vi "picoquant_enqueue_loop_queue.vi"(8 "error in (no error)":errorcluster, 10 "element":T1, 11 "picoquant_generic in":refnum<class "picoquant_generic.lvclass">) -> (0 "error out":errorcluster, 3 "picoquant_generic out":refnum<class "picoquant_generic.lvclass">)   [LabVIEW 2015, in "picoquant_generic.lvclass"]
uses:
  picoquant_generic.lvclass
  loop_notifier_tdef.ctl
  picoquant_generic.lvclass/picoquant_generic.ctl
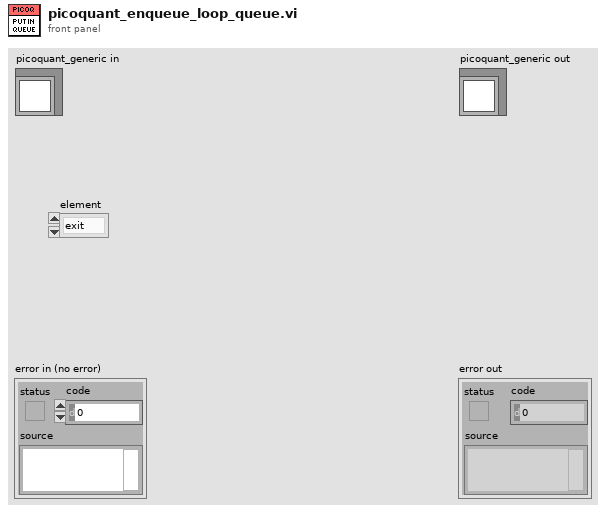
[diagram p1: front panel]
types:
  T1 = typedef "loop_notifier_tdef.ctl" = enum16{"exit"}
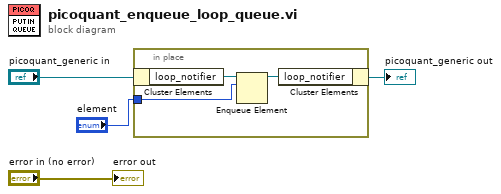
[diagram p0: block diagram]
diagram:
  n1 = in-place {
    in-place-border: "element" -> [w5]
    n2 = in-place-cluster #1("picoquant_generic in") -> ("loop_notifier"=w7:refnum<queue>)
    n3 = Enqueue Element(queue=w7, element=w5) -> (queue out=w6:refnum<queue>)  [unwired: 2 in, 2 out]
    n4 = in-place-cluster #1("loop_notifier"=w6) -> (→"picoquant_generic out":refnum<class "picoquant_generic.lvclass">)
  }
  "error out" <- "error in (no error)"
